vi "Climber_Teleop.vi"(1 "Joystick_Out":T1) -> ()   [LabVIEW 2020]
uses:
  Subsystems/Climber/Climber_Control_States.ctl
  Subsystems/Climber/Climber_Cluster.ctl
  Globals/Climber_Globals.vi
  Utility VIs/Joystick_Controls.ctl
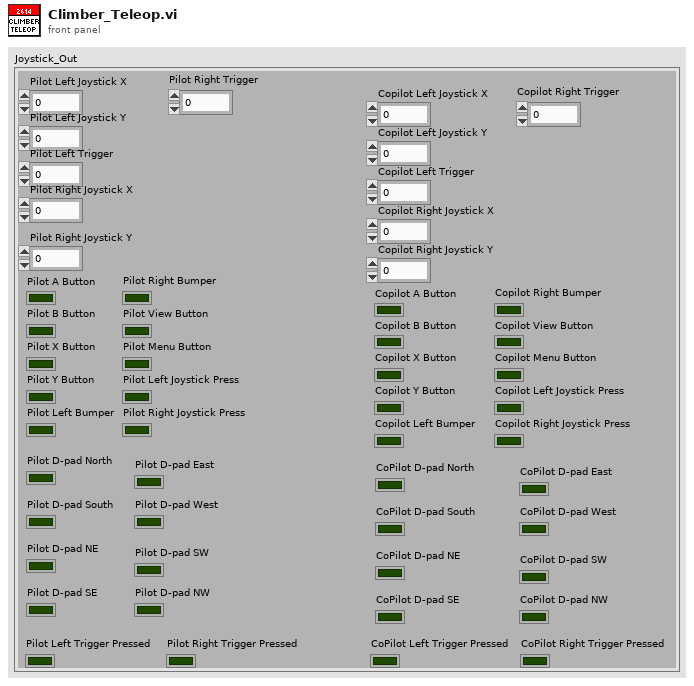
[diagram p1: front panel]
types:
  T1 = typedef "Joystick_Controls.ctl" = cluster{"Pilot Left Joystick X":dbl, "Pilot Left Joystick Y":dbl, "Pilot A Button":bool, "Pilot B Button":bool, "Pilot X Button":bool, "Pilot Y Button":bool, "Pilot Left Bumper":bool, "Pilot Right Bumper":bool, "Pilot View Button":bool, "Pilot Menu Button":bool, "Pilot Left Joystick Press":bool, "Pilot Right Joystick Press":bool, "Pilot Left Trigger":dbl, "Pilot Right Joystick X":dbl, "Pilot Right Joystick Y":dbl, "Pilot Right Trigger":dbl, "Copilot Left Joystick X":dbl, "Copilot Left Joystick Y":dbl, "Copilot A Button":bool, "Copilot B Button":bool, "Copilot X Button":bool, "Copilot Y Button":bool, "Copilot Left Bumper":bool, "Copilot Right Bumper":bool, "Copilot View Button":bool, "Copilot Menu Button":bool, "Copilot Left Joystick Press":bool, "Copilot Right Joystick Press":bool, "Copilot Left Trigger":dbl, "Copilot Right Joystick X":dbl, "Copilot Right Joystick Y":dbl, "Copilot Right Trigger":dbl, "Pilot D-pad North":bool, "Pilot D-pad South":bool, "Pilot D-pad East":bool, "Pilot D-pad West":bool, "Pilot D-pad NE ":bool, "Pilot D-pad SE":bool, "Pilot D-pad SW":bool, "Pilot D-pad NW":bool, "CoPilot D-pad North":bool, "CoPilot D-pad South":bool, "CoPilot D-pad East":bool, "CoPilot D-pad West":bool, "CoPilot D-pad NE":bool, "CoPilot D-pad SE":bool, "CoPilot D-pad SW":bool, "CoPilot D-pad NW":bool, "Pilot Left Trigger Pressed":bool, "Pilot Right Trigger Pressed":bool, "CoPilot Left Trigger Pressed":bool, "CoPilot Right Trigger Pressed":bool}
  T2 = typedef "Climber_Cluster.ctl" = cluster{"Control_State":T3, "Outer_Arm_Pivot_Throttle":dbl, "Outer_Arm_Elevator_Throttle":dbl, "Inner_Arm_Pivot_Throttle":dbl, "Enable_Climber_Sequence":bool}
  T3 = typedef "Climber_Control_States.ctl" = enum16{"No-Op", "Manual_%Vbus", "Climbing_Sequence"}
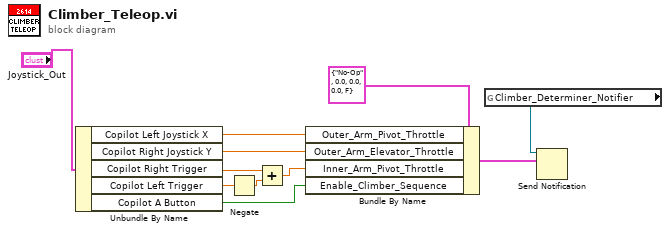
[diagram p0: block diagram]
diagram:
  n1 = Unbundle By Name("Joystick_Out") -> ("Copilot Left Joystick X"=w3:dbl, "Copilot Right Joystick Y"=w4:dbl, "Copilot Right Trigger"=w5:dbl, "Copilot Left Trigger"=w6:dbl, "Copilot A Button"=w9:bool)
  n2 = Negate(x=w6) -> (-x=w7:dbl)
  n3 = Add(x=w5, y=w7) -> (x+y=w8:dbl)
  n4 = Bundle By Name(cluster=T2 {"Control_State"=enum."No-Op", "Outer_Arm_Pivot_Throttle"=0.0, "Outer_Arm_Elevator_Throttle"=0.0, "Inner_Arm_Pivot_Throttle"=0.0, "Enable_Climber_Sequence"=FALSE} ("Climber_Cluster"), "Outer_Arm_Pivot_Throttle"=w3, "Outer_Arm_Elevator_Throttle"=w4, "Inner_Arm_Pivot_Throttle"=w8, "Enable_Climber_Sequence"=w9) -> (w10:T2)
  n5 = global read "Climber_Globals.vi" "Climber_Determiner_Notifier"() -> (w11:refnum<notifier>)
  n6 = Send Notification(notification=w10, notifier=w11) -> ()  [unwired: 1 in, 2 out]
